vi "限幅器（U64）.vi"(3 "下限":u64, 4 "X_in":u64, 5 "上限":u64) -> (1 "X_Out":u64)   [LabVIEW 2012]
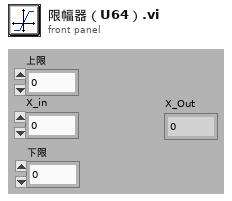
[diagram p1: front panel]
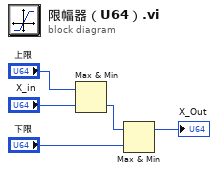
[diagram p0: block diagram]
diagram:
  n1 = Max & Min(x="上限", y="X_in") -> (min(x,y)=w3:u64)  [unwired: 1 out]
  n2 = Max & Min(x=w3, y="下限") -> (max(x,y)=→"X_Out":u64)  [unwired: 1 out]
